vi "FGV T90 Result.vi"(6 "Aktion":enum16{"lesen", "schreiben"}(ring), 11 "T90 Cluster in":T1) -> (3 "T90 Cluster out":T1)   [LabVIEW 2020, in "T90.lvlib"]
uses:
  T90.lvlib
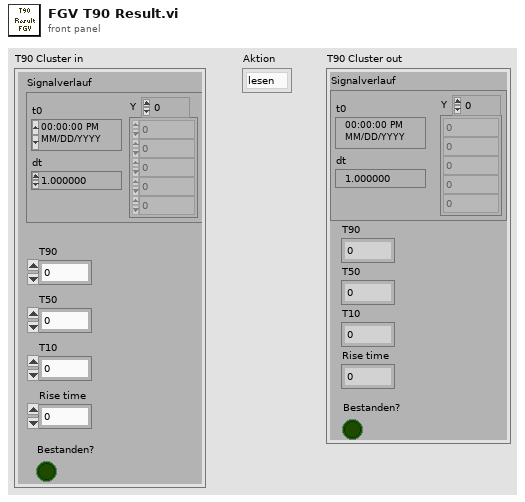
[diagram p1: front panel]
types:
  T1 = cluster{"Signalverlauf":waveform(sgl), "T90":dbl, "T50":dbl, "T10":dbl, "Rise time ":dbl, "Bestanden?":bool}
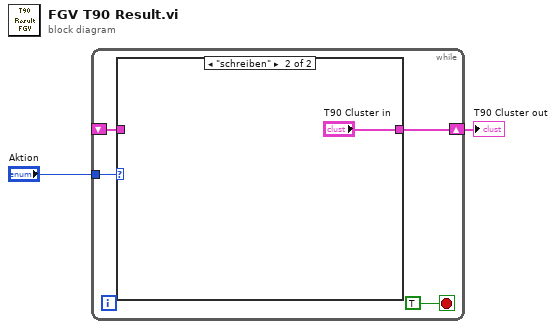
[diagram p0: block diagram]
diagram:
  n1 = while {
    tunnel: "Aktion" -> [w5]
    shift-right: [w4] -> w1
    shift-left: _ -> [w3]
    stop <- TRUE stop-if-true
    n2 = case shown="\"schreiben\"" w5 {
      tunnel: [w7 "T90 Cluster in"] -> w4
      tunnel: w3 -> [w7 _]
      frame "lesen", Default {
      }
      frame "schreiben" {
      }
    }
  }
  "T90 Cluster out" <- w1
